vi "timetest5.vi"() -> ()   [LabVIEW 2015]
uses:
  BERTTA.dll
panel:
  in  "Tcurrent":dbl
  in  "Tset":dbl=100.0
  out "double precision float":dbl
  out "element 7":i32
  out "return type":dbl
  in  "direction":i32
  out "element 6":i32
  in  "rt":i32=60
  out "element 5":i32
  out "element 4":i32
  out "element 3":i32
  out "element 2":i32
  out "element":i32
  in  "pause":i32
  in  "start":i32
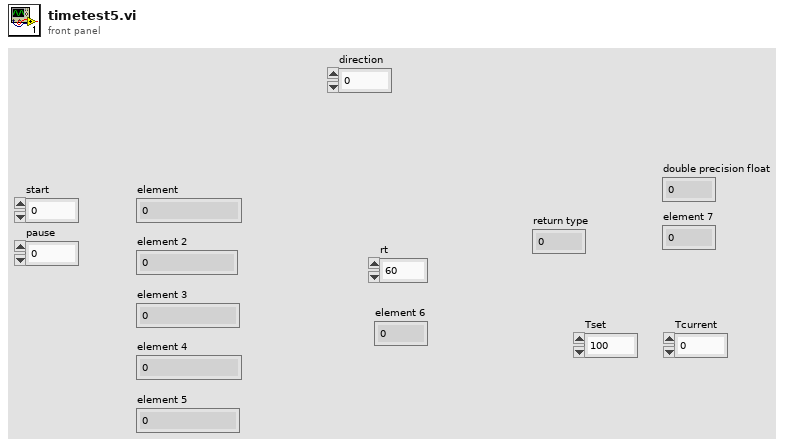
[diagram p1: front panel]
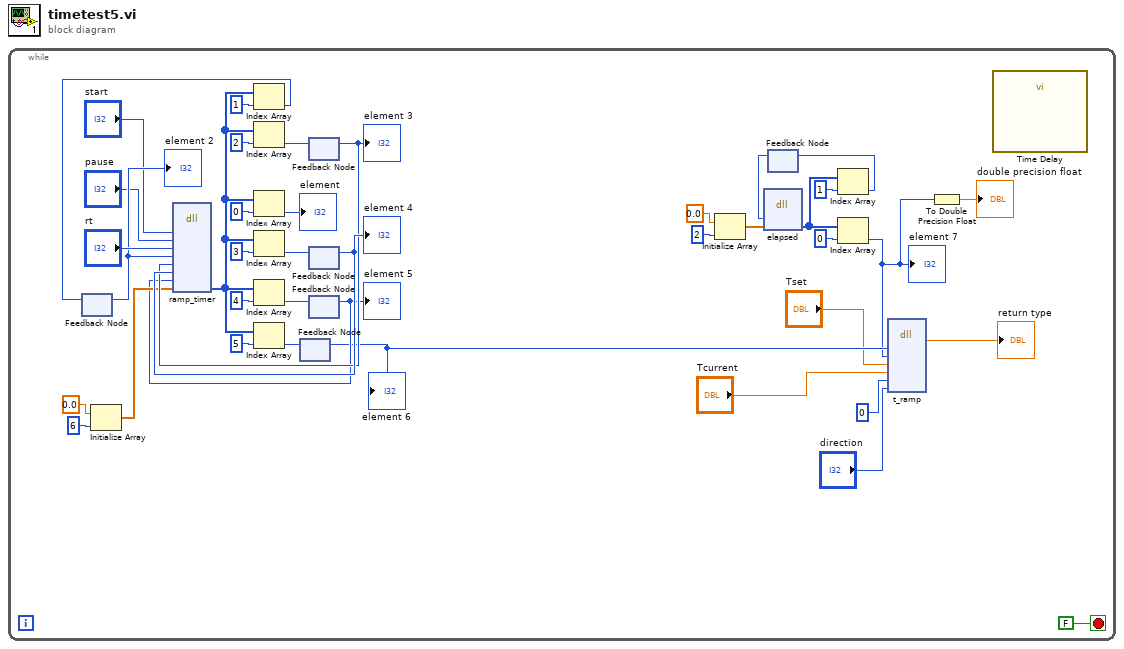
[diagram p0: block diagram]
diagram:
  n1 = while {
    stop <- FALSE stop-if-true
    n2 = feedback #1() -> (w29:i32)  [unwired: 1 in]
    "element 2" <- w29
    n3 = Initialize Array(0.0 ("element"), 6 ("dimension size")) -> (w21:dbl[])
    n4 = feedback #2() -> ()  [unwired: 2 in]
    n5 = feedback #3() -> (w31:i32)  [unwired: 1 in]
    "element 3" <- w31
    n6 = feedback #4() -> (w34:i32)  [unwired: 1 in]
    "element 4" <- w34
    n7 = feedback #5() -> (w18:i32)  [unwired: 1 in]
    "element 5" <- w18
    n8 = dll-call lib="C:/Users/xlaraser/Documents/Visual Studio 2017/Projects/Bertta/BERTTA/Debug/BERTTA.dll" fn="ramp_timer"("enable"="start", "pause"="pause", "rt"="rt", "start_time"=w29, "pause_time"=w31, "paused"=w34, "paused_old"=w18, "params"=w21) -> ("params"=w39:i32[])  [unwired: 11 in, 2 out]
    n9 = Index Array(array=w39, index=1) -> (element=w28:i32)
    n10 = feedback-in #1(w28) -> ()
    n11 = Index Array(array=w39, index=2) -> (element=w30:i32)
    n12 = Index Array(array=w39, index=0) -> (element=→"element":i32)
    n13 = Index Array(array=w39, index=3) -> (element=w33:i32)
    n14 = Index Array(array=w39, index=4) -> (element=w36:i32)
    n15 = Index Array(array=w39, index=5) -> (element=w7:i32)
    "element 6" <- w7
    n16 = feedback-in #2(w7) -> ()
    n17 = feedback-in #3(w30) -> ()
    n18 = feedback-in #4(w33) -> ()
    n19 = feedback-in #5(w36) -> ()
    n20 = Initialize Array(0.0 ("element"), 2 ("dimension size")) -> (w15:dbl[])
    n21 = feedback #6() -> (w8:i32)  [unwired: 1 in]
    n22 = dll-call lib="C:/Users/xlaraser/Documents/Visual Studio 2017/Projects/Bertta/BERTTA/Debug/BERTTA.dll" fn="elapsed"("last_time"=w8, "params"=w15) -> ("params"=w11:i32[])  [unwired: 5 in, 2 out]
    n23 = Index Array(array=w11, index=1) -> (element=w9:i32)
    n24 = feedback-in #6(w9) -> ()
    n25 = Index Array(array=w11, index=0) -> (element=w5:i32)
    "element 7" <- w5
    n26 = dll-call lib="C:/Users/xlaraser/Documents/Visual Studio 2017/Projects/Bertta/BERTTA/Debug/BERTTA.dll" fn="t_ramp"("ramp_time"=w7, "elapsed"=w5, "Tset"="Tset", "Tcurrent"="Tcurrent", "rt"=0, "direction"="direction") -> ("return type"=→"return type":dbl)  [unwired: 9 in, 2 out]
    n27 = To Double Precision Float(number=w5) -> (double precision float=→"double precision float":dbl)
    n28 = call "Time Delay"() -> ()  [unwired: 11 in, 1 out]
  }
